vi "PDF Protokoll T90.vi"(8 "error in (no error)":errorcluster caption="Fehler (Eingang, kein Fehler)") -> (0 "error out":errorcluster caption="Fehler (Ausgang)")   [LabVIEW 2020, in "T90.lvlib"]
uses:
  T90.lvlib
  Zustand Auswahl.ctl
  Aktion FGV T90.ctl
  Seiten/Gaszuordnung AO/FGV Gaszuordnung Grenzen&Einheit Aktion.ctl
  Seiten/FT-IR/FGV FT-IR Gasliste Aktionen.ctl
  Sprachverwaltung/FGV Aktion Tabelle zerlegen.ctl
  Seiten/Anlagengrenzwerte/FGV Anlagengrenzwerte Aktionen.ctl
  <vilib>/Utility/miscctls.llb/LVPrintingMarginsTypeDef.ctl
  Allgemein/allgemeine Sub-VIs.lvlib
  Seiten/FT-IR/FT-IR.lvlib
  Seiten/Gaszuordnung AO/Gaszuordnung AO.lvlib
  Sprachverwaltung/Sprachverwaltung.lvlib
  Seiten/Anlagengrenzwerte/Anlagengrenzwerte.lvlib
panel:
  out "Einheit 2":string caption="Einheit"
  out "Durchfluss FT-IR:":string caption="Fluss FTIR:"
  out "Ergebnis":string caption="Auswertung:"
  out "T90 3":waveform(sgl)(graph) caption="T90"
  out "T90 2":waveform(sgl)(graph) caption="T90"
  out "Abschaltzeit":string caption="Abschaltzeit:"
  out "Rise Time:":string caption="T10 - T90 (Rise Time):"
  out "T10":string caption="T10 (Delay Time):"
  out "T50":string caption="T50 (Response Time):"
  out "T90":string caption="T90 (Response Time):"
  out "Einheit":string
  out "Konzentration:":string
  out "Komponente:":string
  out "Abweichung:":string caption="Abweichung %:"
  out "Modus:":string
  in  "Modus: Ring":T1=1 caption="Modus:" items=["Cal Gas", "Samplepoint"]
  out "T90":waveform(sgl)(graph)
  # "T90 Test"
  # "IAG-Industrie Automatisierungsgeschellschaft m.b.H.    l  Industriestraße 2    l    2722Weikersdorf     )+43262221734 7+43262221734655"
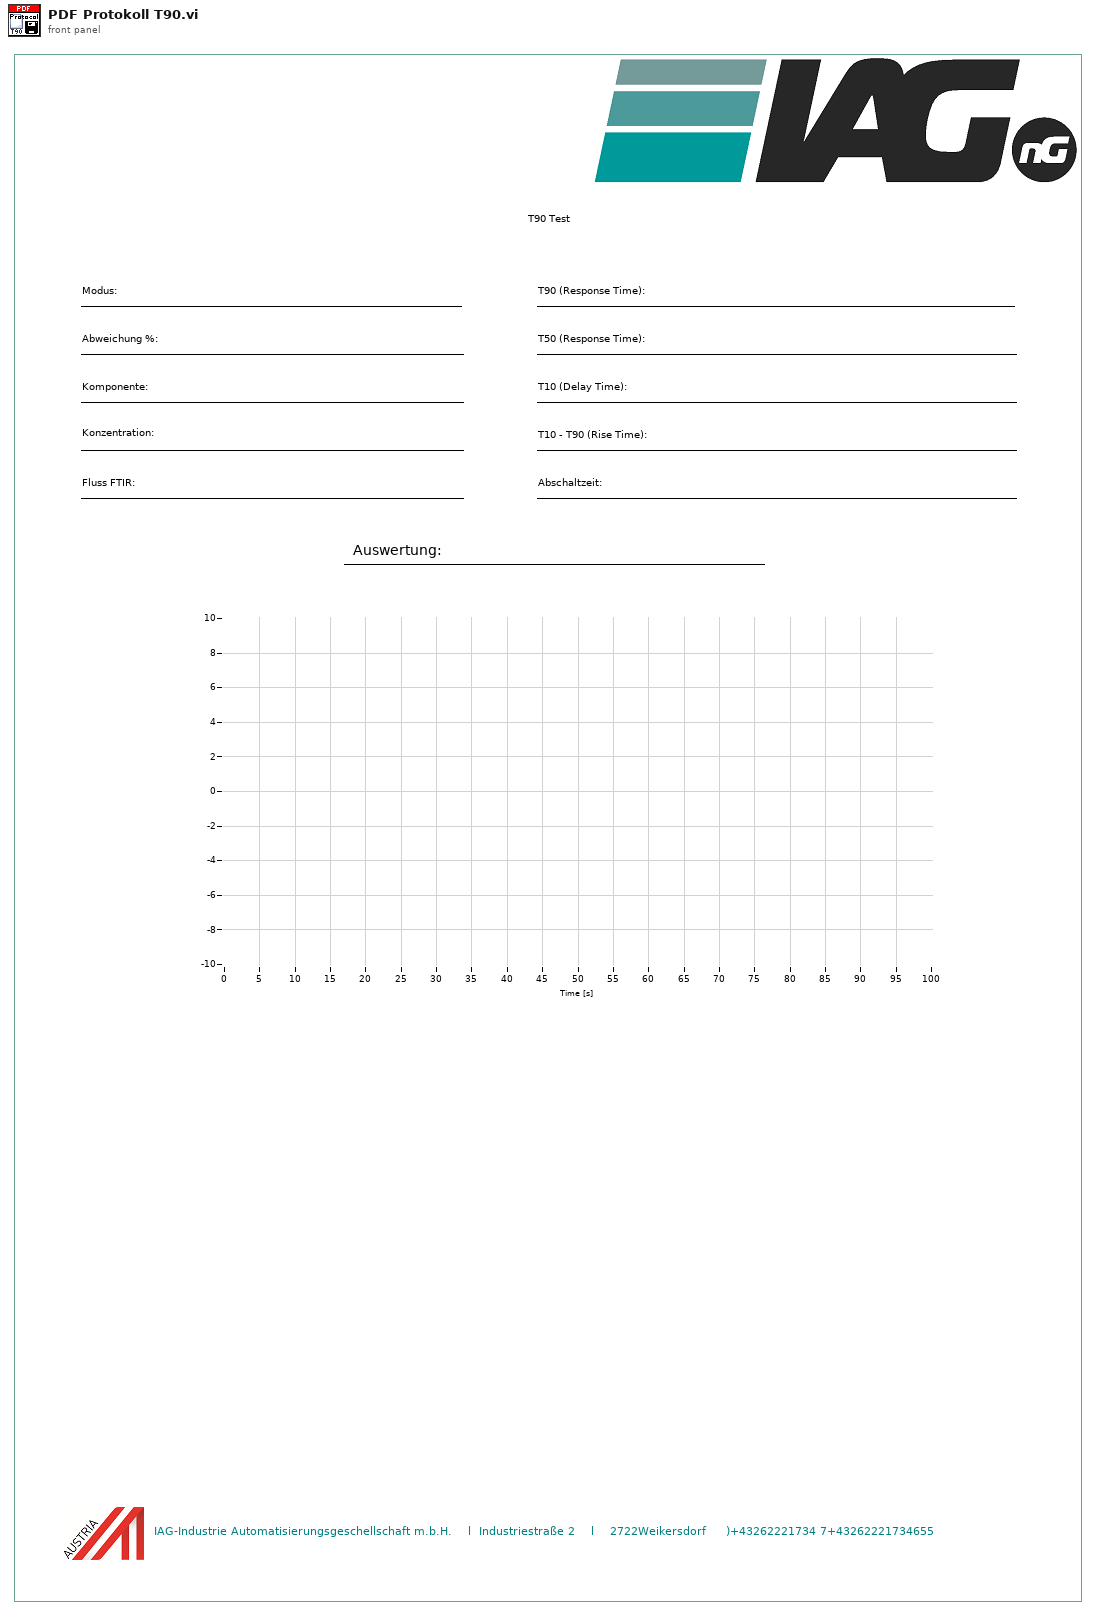
[diagram p1: front panel]
types:
  T1 = typedef "T90.lvlib/Zustand Auswahl.ctl" = u16
  T2 = typedef "Sprachverwaltung.lvlib/FGV Aktion Tabelle zerlegen.ctl" = enum16{"laden", "vereinzeln", "speichern"}
  T3 = typedef "FT-IR.lvlib/FGV FT-IR Gasliste Aktionen.ctl" = enum16{"lesen", "Gasliste FT-IR", "Gasliste ausgelesen", "laden", "speichern", "löschen"}
  T4 = typedef "Gaszuordnung AO.lvlib/FGV Gaszuordnung Grenzen&Einheit Aktion.ctl" = enum16{"Lesen", "Schreiben Min", "Schreiben Max", "Laden", "Speichern"}
  T5 = typedef "T90.lvlib/Aktion FGV T90.ctl" = enum16{"lesen", "schreiben", "laden", "speichern", "T90 aktiv", "T90 Entnahme aktiv", "Overflow Leak", "Pfad", "Zustand", "max. Responsetime"}
  T6 = typedef "Anlagengrenzwerte.lvlib/FGV Anlagengrenzwerte Aktionen.ctl" = enum16{"Lesen", "Grenzwerte schreiben"}
  T7 = enum32{"Portrait", "Landscape", "Rotated Portrait", "Rotated Landscape"}
  T8 = typedef "LVPrintingMarginsTypeDef.ctl" = cluster{"Top":sgl, "Left":sgl, "Bottom":sgl, "Right":sgl, "Measurement System":enum8{"Inches", "cm"}}
  T9 = typedef "T90.lvlib/T90 Gas Konfig.ctl" = cluster{"Gasflasche":T10, "Konfig Gasflasche":T11, "Auswahl":T12, "Sollwert":T13, "Abweichung":T13, "max. Responsetime":T13, "Modus:":T1, "Abschaltzeit":T13, "Stabilisierungszeit":T13, "Bearbeiter":string}
  T10 = typedef "System Einstellungen V2.lvlib/Gasflasche Auswahl.ctl" = u16
  T11 = typedef "System Einstellungen V2.lvlib/Konfig Gasflasche.ctl" = bool
  T12 = typedef "Auswahlfeld.ctl" = u16
  T13 = typedef "Zahlen-Eingabefeld.ctl" = sgl
  T14 = typedef "Anlagengrenzwerte.lvlib/Anlagen-Grenzwerte Anzeige.ctl" = cluster{"Eingangsdruck FT-IR:":T15, "Durchfluss FT-IR:":T15, "Durchfluss CalGas:":T15, "Druck Ausgang:":T15, "Druck Kalter Block:":T15, "Heizleitungen intern:":T15, "Heizleitung zu FT-IR:":T15, "Heizung Filterblock:":T15, "Heizung Pumpe:":T15, "Heizleitung Extern SP1:":T15, "Heizleitung Extern SP2:":T15, "FT-IR Heizung Messzelle:":T15, "Schaltschranktemperatur:":T15, "Gaskühler:":T15}
  T15 = typedef "Anlagengrenzwerte.lvlib/Anlagen-Parameter Anzeige.ctl" = cluster{"Sollwert":sgl, "Warn-Min":sgl, "Warn-Max":sgl, "Abschalt-Min":sgl, "Abschalt-Max":sgl, "Regler":u16}
  T16 = typedef "String - Ausgabefeld.ctl" = string
  T17 = cluster{"Signalverlauf":waveform(sgl), "T90":dbl, "T50":dbl, "T10":dbl, "Rise time ":dbl, "Bestanden?":bool}
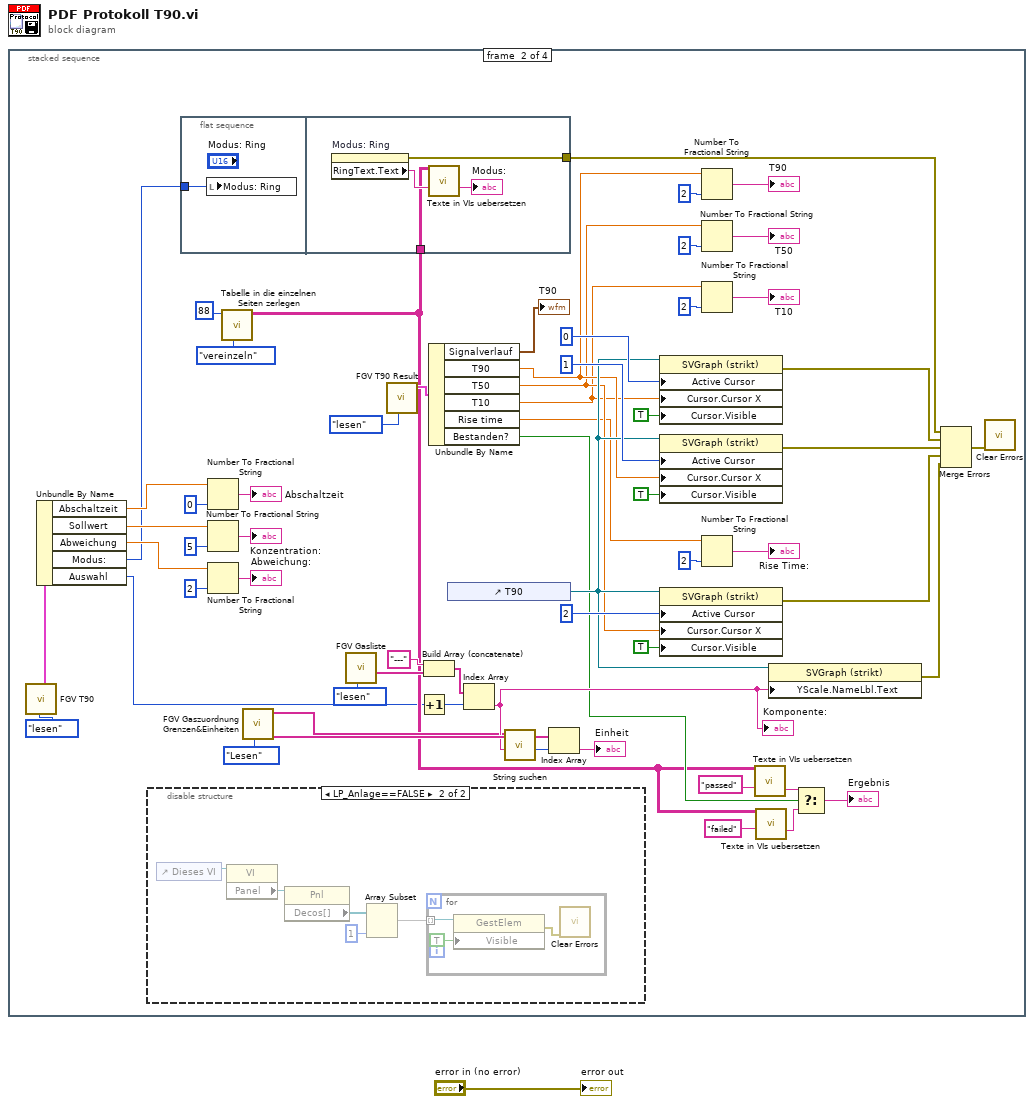
[diagram p0: block diagram]
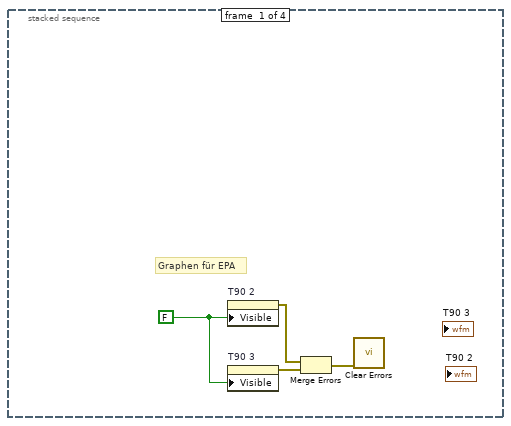
[diagram p2: hidden frame]
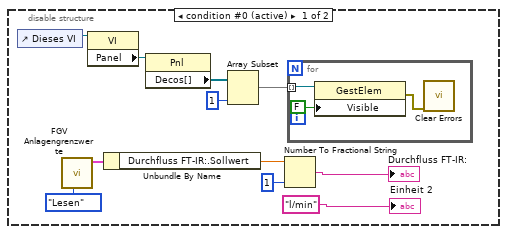
[diagram p3: hidden frame]
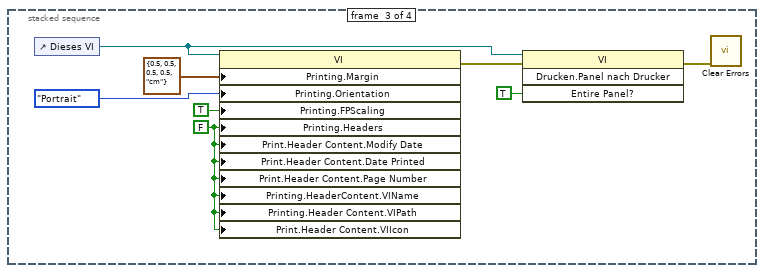
[diagram p4: hidden frame]
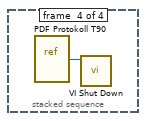
[diagram p5: hidden frame]
diagram:
  n1 = stacked-sequence {
    frame #0 {
      w5 = FALSE
      # "Graphen für EPA"
      n2 = property on="T90 2" class="SVGraph (strikt)"("Visible"=w5) -> (error out=w3:errorcluster)  [unwired: 2 in, 1 out]
      n3 = property on="T90 3" class="SVGraph (strikt)"("Visible"=w5) -> (error out=w2:errorcluster)  [unwired: 2 in, 1 out]
      n4 = Merge Errors(w3, w2) -> (w4:errorcluster)
      n5 = call <vilib>:"Clear Errors.vi"("error in (no error)"=w4) -> ()  [unwired: 5 in, 2 out]
    }
    frame #1 {
      n6 = call "FGV T90.vi"("Aktion"=Aktion_FGV_T90."lesen") -> ("Gas Konfig"=w19:T9)  [unwired: 20 in, 6 out]
      n7 = Unbundle By Name(w19) -> ("Abschaltzeit"=w18:T13, "Sollwert"=w17:T13, "Abweichung"=w16:T13, "Modus:"=w15:T1, "Auswahl"=w7:T12)
      n8 = disable-structure shown="LP_Anlage==FALSE" {
        frame condition #0 (active) {
          n9 = control-ref of="Dieses VI"() -> (w73:refnum<vi>)
          n10 = call "FGV Anlagengrenzwerte.vi"("Aktion"=FGV_Anlagengrenzwerte_Aktionen."Lesen") -> ("Anlagen-Grenzwerte Anzeige"=w75:T14)  [unwired: 1 in, 9 out]
          n11 = property class="VI"(reference=w73) -> ("Panel"=w70:refnum<vi>)  [unwired: 1 in, 2 out]
          n12 = Unbundle By Name(w75) -> ("Durchfluss FT-IR:.Sollwert"=w74:sgl)
          n13 = property class="Pnl"(reference=w70) -> ("Decos[]"=w71:refnum<vi>[])  [unwired: 1 in, 2 out]
          n14 = Array Subset(array=w71, length=1 ("Länge")) -> (w72:refnum<vi>[])  [unwired: 1 in]
          n15 = Number To Fractional String(number=w74, precision (6)=i16 1 ("Genauigkeit (6)")) -> (F-format string=→"Durchfluss FT-IR:":string)  [unwired: 2 in]
          n16 = for {
            tunnel: w72 -> [w80] mode=indexing
            n17 = property class="GestElem"(reference=w80, "Visible"=FALSE ("Sichtbar")) -> (error out=w78:errorcluster)  [unwired: 1 in, 1 out]
            n18 = call <vilib>:"Clear Errors.vi"("error in (no error)"=w78) -> ()  [unwired: 5 in, 2 out]
          }
          "Einheit 2" <- "l/min" ("Einheit 2")
        }
        frame condition #1 {
          n19 = control-ref of="Dieses VI"() -> (w85:refnum<vi>)
          n20 = property class="VI"(reference=w85) -> ("Panel"=w82:refnum<vi>)  [unwired: 1 in, 2 out]
          n21 = property class="Pnl"(reference=w82) -> ("Decos[]"=w83:refnum<vi>[])  [unwired: 1 in, 2 out]
          n22 = Array Subset(array=w83, length=1 ("Länge")) -> (w84:refnum<vi>[])  [unwired: 1 in]
          n23 = for {
            tunnel: w84 -> [w88] mode=indexing
            n24 = property class="GestElem"(reference=w88, "Visible"=TRUE ("Sichtbar")) -> (error out=w86:errorcluster)  [unwired: 1 in, 1 out]
            n25 = call <vilib>:"Clear Errors.vi"("error in (no error)"=w86) -> ()  [unwired: 5 in, 2 out]
          }
        }
      }
      n26 = flat-sequence {
        tunnel: w15 -> [w89]
        tunnel: [w93] -> w30
        tunnel: w8 -> [w90]
        frame #0 {
          n27 = local write "Modus: Ring"(w89) -> ()
        }
        frame #1 {
          n28 = property on="Modus: Ring" class="Ring (strikt)"() -> (error out=w93:errorcluster, "RingText.Text"=w92:string)  [unwired: 2 in, 1 out]
          n29 = call "Texte in VIs uebersetzen.vi"("Sprachliste"=w90, "String zum Übersetzen"=w92) -> ("String zum Übersetzen"=→"Modus:":string)  [unwired: 9 in, 4 out]
        }
      }
      n30 = Number To Fractional String(number=w18, precision (6)=i16 0 ("Genauigkeit (6)")) -> (F-format string=→"Abschaltzeit":string)  [unwired: 2 in]
      n31 = Number To Fractional String(number=w17, precision (6)=i16 5 ("Genauigkeit (6)")) -> (F-format string=→"Konzentration:":string)  [unwired: 2 in]
      n32 = Number To Fractional String(number=w16, precision (6)=i16 2 ("Genauigkeit (6)")) -> (F-format string=→"Abweichung:":string)  [unwired: 2 in]
      n33 = call "Tabelle in die einzelnen Seiten zerlegen.vi"("Aktion"=FGV_Aktion_Tabelle_zerlegen."vereinzeln", "Index (Seite)"=88) -> ("Sprachliste"=w8:string[][])  [unwired: 7 in, 2 out]
      n34 = call "FGV Gaszuordnung Grenzen&Einheiten.vi"("Aktion"=FGV_Gaszuordnung_Grenzen&Einheit_Aktion."Lesen") -> ("Einheit neu"=w51:string[], "Namen neu"=w24:string[])  [unwired: 7 in, 2 out]
      n35 = call "FGV Gasliste.vi"("Aktionen"=FGV_FT-IR_Gasliste_Aktionen."lesen") -> ("Aktuelle Gasliste gesamt"=w54:T16[])  [unwired: 8 in, 2 out]
      n36 = call "FGV T90 Result.vi"("Aktion"=enum16{"lesen", "schreiben"}."lesen") -> ("T90 Cluster out"=w45:T17)  [unwired: 10 in]
      n37 = Increment(x=w7) -> (x+1=w6:T12)
      n38 = Build Array (concatenate)("---", w54) -> (w55:T16[])
      n39 = Unbundle By Name(w45) -> ("Signalverlauf"=→"T90":waveform(sgl), "T90"=w38:dbl, "T50"=w37:dbl, "T10"=w36:dbl, "Rise time"=w35:dbl, "Bestanden?"=w21:bool)
      n40 = control-ref of="T90"() -> (w53:refnum<vi>)
      n41 = Index Array(array=w55, index=w6) -> (element=w25:T16)
      "Komponente:" <- w25
      n42 = call "String suchen.vi"("Gasname"=w25, "Such-Namen"=w24) -> ("Index"=w23:i32)  [unwired: 8 in, 1 out]
      n43 = Index Array(array=w51, index=w23) -> (element=→"Einheit":string)
      n44 = property on="Eigenschaftsknoten" class="SVGraph (strikt)"(reference=w53, "Active Cursor"=u32 0 ("Aktiver Cursor"), "Cursor.Cursor X"=w36, "Cursor.Visible"=TRUE ("Cursor.Sichtbar")) -> (error out=w29:errorcluster)  [unwired: 1 in, 1 out]
      n45 = property on="Eigenschaftsknoten" class="SVGraph (strikt)"(reference=w53, "Active Cursor"=u32 1 ("Aktiver Cursor"), "Cursor.Cursor X"=w38, "Cursor.Visible"=TRUE ("Cursor.Sichtbar")) -> (error out=w28:errorcluster)  [unwired: 1 in, 1 out]
      n46 = property on="Eigenschaftsknoten" class="SVGraph (strikt)"(reference=w53, "Active Cursor"=u32 2 ("Aktiver Cursor"), "Cursor.Cursor X"=w37, "Cursor.Visible"=TRUE ("Cursor.Sichtbar")) -> (error out=w27:errorcluster)  [unwired: 1 in, 1 out]
      n47 = Number To Fractional String(number=w38, precision (6)=i16 2 ("Genauigkeit (6)")) -> (F-format string=→"T90":string)  [unwired: 2 in]
      n48 = Number To Fractional String(number=w37, precision (6)=i16 2 ("Genauigkeit (6)")) -> (F-format string=→"T50":string)  [unwired: 2 in]
      n49 = Number To Fractional String(number=w36, precision (6)=i16 2 ("Genauigkeit (6)")) -> (F-format string=→"T10":string)  [unwired: 2 in]
      n50 = Number To Fractional String(number=w35, precision (6)=i16 2 ("Genauigkeit (6)")) -> (F-format string=→"Rise Time:":string)  [unwired: 2 in]
      n51 = call "Texte in VIs uebersetzen.vi"("Sprachliste"=w8, "String zum Übersetzen"="passed") -> ("String zum Übersetzen"=w13:string)  [unwired: 9 in, 4 out]
      n52 = call "Texte in VIs uebersetzen.vi"("Sprachliste"=w8, "String zum Übersetzen"="failed") -> ("String zum Übersetzen"=w12:string)  [unwired: 9 in, 4 out]
      n53 = property on="Eigenschaftsknoten" class="SVGraph (strikt)"(reference=w53, "YScale.NameLbl.Text"=w25) -> (error out=w26:errorcluster)  [unwired: 1 in, 1 out]
      n54 = Select(t=w13, s=w21, f=w12) -> (s? t:f=→"Ergebnis":string)
      n55 = Merge Errors(w30, w29, w28, w27, w26) -> (w59:errorcluster)
      n56 = call <vilib>:"Clear Errors.vi"("error in (no error)"=w59) -> ()  [unwired: 5 in, 2 out]
    }
    frame #2 {
      w97 = FALSE ("Drucken:Kopfzeilen?")
      n57 = control-ref of="Dieses VI"() -> (w94:refnum<vi>)
      n58 = property class="VI"(reference=w94, "Printing.Margin"=T8 {"Top"=0.5, "Left"=0.5, "Bottom"=0.5, "Right"=0.5, "Measurement System"=enum."cm"} ("Drucken:Ränder"), "Printing.Orientation"=T7."Portrait" ("Drucken:Seitenausrichtung"), "Printing.FPScaling"=TRUE ("Drucken:Frontpanel-Skalierung?"), "Printing.Headers"=w97, "Print.Header Content.Modify Date"=w97, "Print.Header Content.Date Printed"=w97, "Print.Header Content.Page Number"=w97, "Printing.HeaderContent.VIName"=w97, "Printing.Header Content.VIPath"=w97, "Print.Header Content.VIIcon"=w97) -> (error out=w101:errorcluster)  [unwired: 1 in, 1 out]
      n59 = invoke class="VI" method="Drucken.Panel nach Drucker"(reference=w94, error in=w101, "Entire Panel?"=TRUE ("Abschnittskopfzeilen?")) -> (error out=w95:errorcluster)  [unwired: 1 in, 3 out]
      n60 = call <vilib>:"Clear Errors.vi"("error in (no error)"=w95) -> ()  [unwired: 5 in, 2 out]
    }
    frame #3 {
      n61 = vi-ref "PDF Protokoll T90.vi"() -> (w102:refnum<vi>)
      n62 = call "VI Shut Down.vi"("VI Referenz"=w102) -> ()  [unwired: 11 in]
    }
  }
  "error out" <- "error in (no error)"
